vi "ContourFilled_Automatic.vi"(4 "Properties":T2={"Colormap"={"Map"=enum."Automatic", "Value Min"=nan, "Value Max"=nan, "Scaling"=enum."Default", "Reverse"=FALSE}, "Display"={"Alpha"=nan, "Z Order"=nan}}, 5 "Levels":i32=-1, 6 "Contour Range":T1={"Min Level"=nan, "Max Level"=nan}, 7 "Z Data":dbl[][](array[numeric]), 8 "error in (no error)":errorcluster, 9 "Y Coordinates":dbl[](array[numeric]), 10 "X Coordinates":dbl[](array[numeric]), 11 "Plot ID":T7 format="%x") -> (0 "error out":errorcluster, 3 "Plot ID Out":T7 format="%x")   [LabVIEW 2013, in "Advanced Plotting Toolkit.lvlib"]
doc: "Generate a filled contour plot, from a specific number of contour levels.\n\nNote this VI does the filled regions only; use Contour.vi for lines."
uses:
  Advanced Plotting Toolkit.lvlib
  typedefs/PlotID.ctl
  ContourFilledProperties.ctl
  properties/Colormap.ctl
  properties/Colormap_Map.ctl
  properties/Colormap_Scaling.ctl
  properties/Display.ctl
  ContourRange.ctl
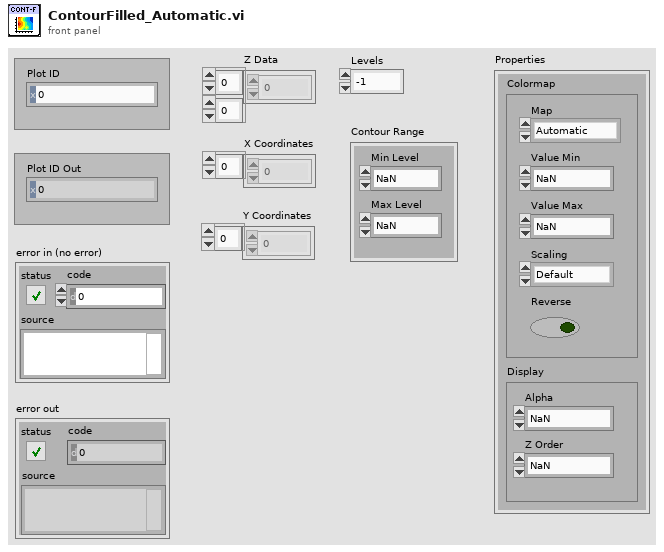
[diagram p1: front panel]
types:
  T1 = typedef "Advanced Plotting Toolkit.lvlib/ContourRange.ctl" = cluster{"Min Level":dbl, "Max Level":dbl}
  T2 = typedef "Advanced Plotting Toolkit.lvlib/ContourFilledProperties.ctl" = cluster{"Colormap":T3, "Display":T6}
  T3 = typedef "Advanced Plotting Toolkit.lvlib/Colormap.ctl" = cluster{"Map":T4, "Value Min":dbl, "Value Max":dbl, "Scaling":T5, "Reverse":bool}
  T4 = typedef "Advanced Plotting Toolkit.lvlib/Colormap_Map.ctl" = enum16{"Automatic", "Rainbow", "Hot and Cold", "White-Black", "White-Blue", "White-Green", "White-Red", "Fire", "Water", "Earth", "Air", "Pastel", "Banded", "Stepped"}
  T5 = typedef "Advanced Plotting Toolkit.lvlib/Colormap_Scaling.ctl" = enum16{"Default"}
  T6 = typedef "Advanced Plotting Toolkit.lvlib/Display.ctl" = cluster{"Alpha":dbl, "Z Order":dbl}
  T7 = typedef "Advanced Plotting Toolkit.lvlib/PlotID.ctl" = i32
  T8 = typedef "Advanced Plotting Toolkit.lvlib/KeyValue.ctl" = cluster{"Key":string, "Value":string}
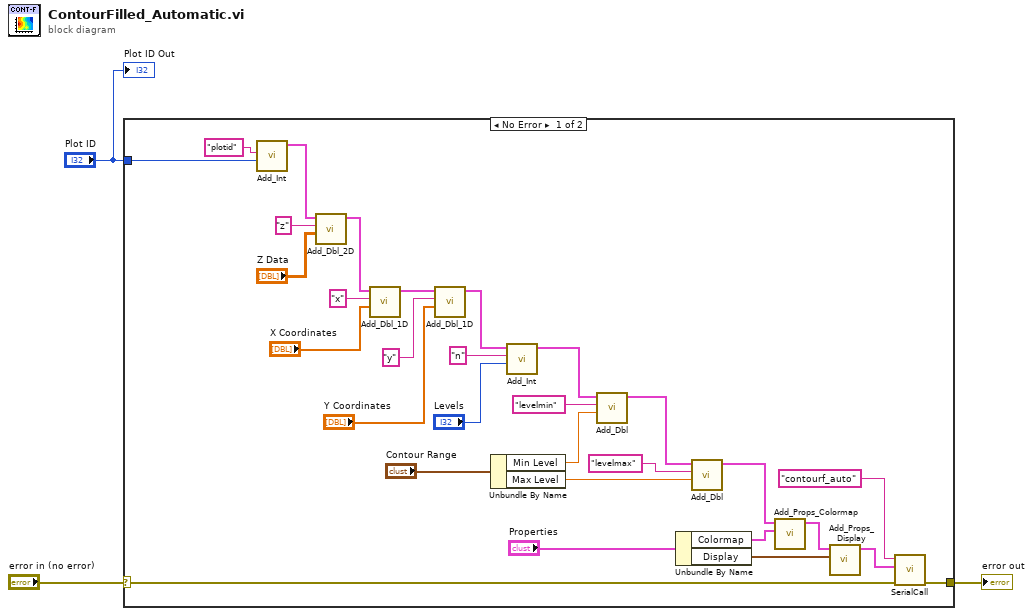
[diagram p0: block diagram]
diagram:
  n1 = case shown="No Error" "error in (no error)" {
    selector: "error in (no error)" -> [w22 w34]
    tunnel: "Plot ID" -> [w20 _]
    tunnel: [w21 w34] -> w1
    frame No Error {
      n2 = call "Add_Int.vi"("Value"=w20, "Key"="plotid") -> ("Keyword Array Out"=w28:T8[])  [unwired: 9 in]
      n3 = call "Add_Dbl_2D.vi"("Value"="Z Data", "Key"="z", "Keyword Array"=w28) -> ("Keyword Array Out"=w27:T8[])  [unwired: 8 in]
      n4 = call "Add_Dbl_1D.vi"("Value"="X Coordinates", "Key"="x", "Keyword Array"=w27) -> ("Keyword Array Out"=w26:T8[])  [unwired: 8 in]
      n5 = call "Add_Dbl_1D.vi"("Value"="Y Coordinates", "Key"="y", "Keyword Array"=w26) -> ("Keyword Array Out"=w25:T8[])  [unwired: 8 in]
      n6 = Unbundle By Name("Contour Range") -> ("Min Level"=w9:dbl, "Max Level"=w7:dbl)
      n7 = call "Add_Int.vi"("Value"="Levels", "Key"="n", "Keyword Array"=w25) -> ("Keyword Array Out"=w6:T8[])  [unwired: 8 in]
      n8 = call "Add_Dbl.vi"("Value"=w9, "Key"="levelmin", "Keyword Array"=w6) -> ("Keyword Array Out"=w5:T8[])  [unwired: 8 in]
      n9 = Unbundle By Name("Properties") -> ("Colormap"=w14:T3, "Display"=w12:T6)
      n10 = call "Add_Dbl.vi"("Value"=w7, "Key"="levelmax", "Keyword Array"=w5) -> ("Keyword Array Out"=w4:T8[])  [unwired: 8 in]
      n11 = call "Add_Props_Colormap.vi"("Colormap"=w14, "Keyword Array"=w4) -> ("Keyword Array Out"=w13:T8[])  [unwired: 9 in]
      n12 = call "Add_Props_Display.vi"("Display"=w12, "Keyword Array"=w13) -> ("Keyword Array Out"=w15:T8[])  [unwired: 9 in]
      n13 = call "SerialCall.vi"("error in (no error)"=w22, "data"=w15, "Resource"="contourf_auto") -> ("error out"=w21:errorcluster)  [unwired: 7 in, 1 out]
    }
    frame Error {
    }
  }
  "error out" <- w1
  "Plot ID Out" <- "Plot ID"
